vi "SecBiopLoc.vi"(6 "Ref Sector EndPts":T2={"x1"=453.0, "y1"=119.0, "x2"=453.0, "y2"=306.0, "x3"=463.0, "y3"=119.0, "x4"=463.0, "y4"=119.0} {"y4" format="%.2f"; "x4" format="%.2f"; "y3" format="%.2f"; "x3" format="%.2f"; "y2" format="%.2f"; "x2" format="%.2f"; "y1" format="%.2f"; "x1" format="%.2f"}, 7 "start path":path) -> (0 "Sector Endpts out":T1(array[cluster]) {"y4" format="%.2f"; "x4" format="%.2f"; "y3" format="%.2f"; "x3" format="%.2f"; "y2" format="%.2f"; "x2" format="%.2f"; "y1" format="%.2f"; "x1" format="%.2f"}, 2 "Listbox":i32[](array[numeric]), 3 "File names":string[](array[string]))   [LabVIEW 2022 SP3]
panel:
  out "Waveform Graph":dbl[](graph)
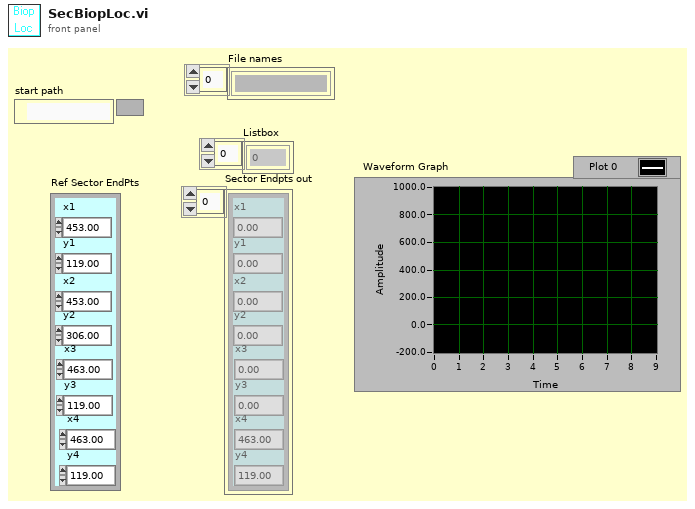
[diagram p1: front panel]
types:
  T1 = cluster{"x1":dbl, "y1":dbl, "x2":dbl, "y2":dbl, "x3":dbl, "y3":dbl, "x4":dbl, "y4":dbl}[]
  T2 = cluster{"x1":dbl, "y1":dbl, "x2":dbl, "y2":dbl, "x3":dbl, "y3":dbl, "x4":dbl, "y4":dbl}
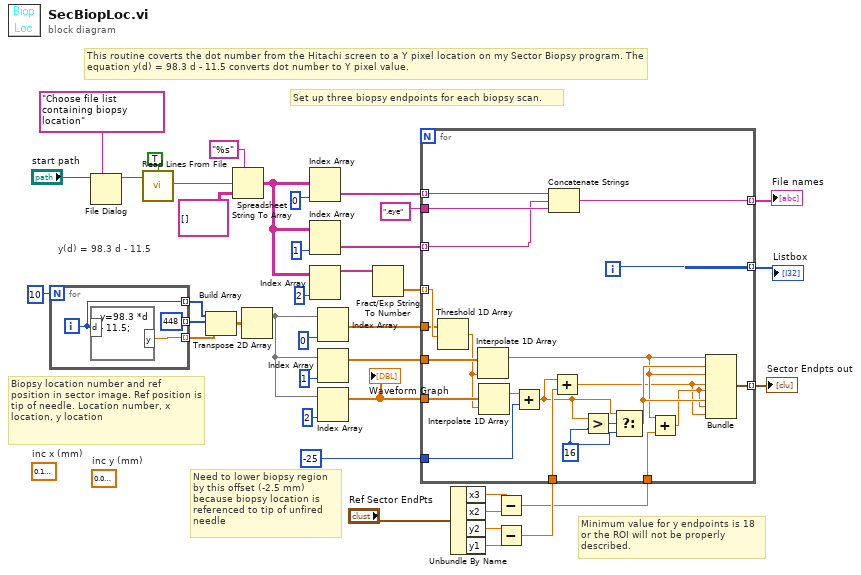
[diagram p0: block diagram]
diagram:
  (unwired) 0.0970304031824913  # inc y (mm)
  (unwired) 0.1553949140240016  # inc x (mm)
  # "This routine coverts the dot number from the Hitachi screen to a Y pixel location on my Sector Biopsy program. The equation y(d) = 98.3 d - 11.5 converts dot number to Y pixel value."
  # "Minimum value for y endpoints is 18 or the ROI will not be properly described."
  # "y(d) = 98.3 d - 11.5"
  # "Set up three biopsy endpoints for each biopsy scan."
  # "Need to lower biopsy region by this offset (-2.5 mm) because biopsy location is referenced to tip of unfired needle"
  # "Biopsy location number and ref position in sector image. Ref position is tip of needle. Location number, x location, y location"
  n1 = for {
    N: 10 -> [_]
    tunnel: [w42] -> w8 mode=indexing
    tunnel: [w41] -> w6 mode=indexing
    tunnel: [448] -> w7 mode=indexing
    i -> [w42]
    n2 = formula code="y=98.3 *d - 11.5;"("d"=w42) -> ("y"=w41:dbl)
  }
  n3 = File Dialog(7:"Choose file list containing biopsy location" ("prompt"), 11:"start path") -> (3:w35:path)  [unwired: 1 in, 7 out]
  n4 = call <vilib>:"Read Lines From File.vi"("convert eol? (no:F)"=TRUE, "file path (dialog if empty)"=w35) -> ("line string"=w39:string)  [unwired: 1 in, 6 out]
  n5 = Build Array(w8, w7, w6) -> (w5:dbl[][])
  n6 = Spreadsheet String To Array(format string="%s", spreadsheet string=w39, array type (2D Dbl)=string[][] [] ("Array Constant")) -> (array=w24:string[][])  [unwired: 1 in]
  n7 = Transpose 2D Array(2D array=w5) -> (transposed array=w4:dbl[][])
  n8 = Index Array(array=w24, index (col)=0) -> (element=w23:string[])  [unwired: 1 in]
  n9 = Index Array(array=w24, index (col)=1) -> (element=w22:string[])  [unwired: 1 in]
  n10 = Index Array(array=w24, index (col)=2) -> (element=w15:string[])  [unwired: 1 in]
  n11 = Index Array(array=w4, index (col)=0) -> (element=w3:dbl[])  [unwired: 1 in]
  n12 = Index Array(array=w4, index (col)=1) -> (element=w2:dbl[])  [unwired: 1 in]
  n13 = Index Array(array=w4, index (col)=2) -> (element=w1:dbl[])  [unwired: 1 in]
  "Waveform Graph" <- w1
  n14 = Fract/Exp String To Number(string=w15) -> (number=w14:dbl[])  [unwired: 4 out]
  n15 = Unbundle By Name("Ref Sector EndPts") -> ("x3"=w30:dbl, "x2"=w29:dbl, "y2"=w28:dbl, "y1"=w27:dbl)
  n16 = Subtract(x=w30, y=w29) -> (x-y=w12:dbl)
  n17 = Subtract(x=w28, y=w27) -> (x-y=w13:dbl)
  n18 = for {
    tunnel: w23 -> [w64] mode=indexing
    tunnel: w22 -> [w46] mode=indexing
    tunnel: ".eye" -> [w63]
    tunnel: [w62] -> w20 mode=indexing
    tunnel: [w61] -> w19 mode=indexing
    tunnel: w3 -> [w59]
    tunnel: w2 -> [w58]
    tunnel: w1 -> [w57]
    tunnel: w14 -> [w60] mode=indexing
    tunnel: w13 -> [w55]
    tunnel: w12 -> [w54]
    tunnel: [w53] -> w11 mode=indexing
    tunnel: -25 -> [w51]
    i -> [w61]
    w50 = 16
    n19 = Threshold 1D Array(2:w60, 3:w59) -> (0:w56:dbl)  [unwired: 1 out]
    n20 = Interpolate 1D Array(1:w56, 2:w58) -> (0:w45:dbl)
    n21 = Interpolate 1D Array(1:w56, 2:w57) -> (0:w52:dbl)
    n22 = Add(x=w52, y=w51) -> (x+y=w49:dbl)
    n23 = Concatenate Strings(w64, w46, w63) -> (w62:string)
    n24 = Add(x=w49, y=w55) -> (x+y=w43:dbl)
    n25 = Greater?(x=w49, y=w50) -> (0:w47:bool)
    n26 = Select(t=w49, s=w47, f=w50) -> (s? t:f=w48:dbl)
    n27 = Add(x=w45, y=w54) -> (x+y=w44:dbl)
    n28 = Bundle(w45, w48, w45, w43, w44, w48, w44, w43) -> (w53:cluster{dbl, dbl, dbl, dbl, dbl, dbl, dbl, dbl})  [unwired: 1 out]
  }
  "File names" <- w20
  "Listbox" <- w19
  "Sector Endpts out" <- w11
